vi "Search etc-hosts contents.vi"(8 "error in (no error)":errorcluster, 10 "hostname":string, 11 "/etc/hosts contents":string) -> (0 "error out":errorcluster, 3 "addresses":refnum<class "Generic Network Address.lvclass">[](array[class]))   [LabVIEW 2020, in "NI_WFCN.lvlib" / "Hostname Network Address.lvclass"]
doc: "FInd all definitions of the specified hostname in an already-read-from-disk /etc/hosts file."
uses:
  <vilib>/net/WFCN/Addressing/Hostname Network Address/Hostname Network Address.lvclass
  <vilib>/net/WFCN/Addressing/Generic Network Address/Generic Network Address.lvclass
  <vilib>/net/WFCN/Addressing/IPv4 Network Address/IPv4 Network Address.lvclass/IPv4 Network Address.ctl
  <vilib>/net/WFCN/Addressing/Generic Network Address/Generic Network Address.lvclass/Generic Network Address.ctl
  <vilib>/net/WFCN/Addressing/Hostname Network Address/Hostname Network Address.lvclass/Hostname Network Address.ctl
  <vilib>/net/WFCN/Addressing/Hostname Network Address/Create from string.vi
  <vilib>/net/WFCN/Utility/Is IPv4 address.vi
  <vilib>/net/WFCN/Addressing/IPv4 Network Address/Create from U32.vi
  <vilib>/net/WFCN/Addressing/Generic Network Address/Create for unparsable.vi
  <vilib>/net/WFCN/Utility/Is hostname mDNS.vi
  <vilib>/dlg_ctls.llb/Space Constant.vi
  <vilib>/net/WFCN/Addressing/IPv4 Network Address/IPv4 Network Address.lvclass
  e:/builds/penguin/labview/branches/2020/dev/dist/vi.lib/net/WFCN/Addressing/Generic Network Address/Generic Network Address.lvclass
  <vilib>/net/WFCN/Addressing/mDNS Hostname Network Address/mDNS Hostname Network Address.lvclass
  e:/builds/penguin/labview/branches/2020/dev/dist/vi.lib/net/WFCN/Addressing/Hostname Network Address/Hostname Network Address.lvclass
  <vilib>/Utility/error.llb/Error Cluster From Error Code.vi
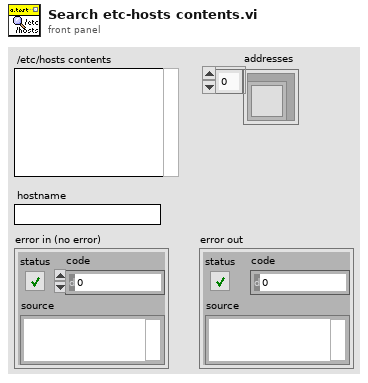
[diagram p1: front panel]
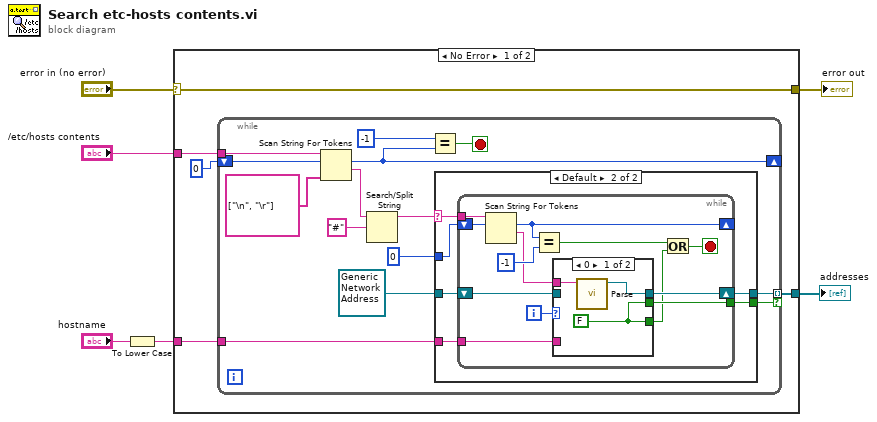
[diagram p0: block diagram]
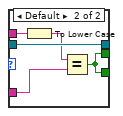
[diagram p3: hidden frame]
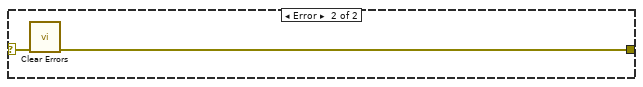
[diagram p4: hidden frame]
diagram:
  n1 = To Lower Case(string="hostname") -> (all lower case string=w1:string)
  n2 = case shown="No Error" "error in (no error)" {
    selector: "error in (no error)" -> [w9 w55]
    tunnel: [w9 w54] -> w4
    tunnel: "/etc/hosts contents" -> [w11 _]
    tunnel: w1 -> [w8 _]
    tunnel: [w7 _] -> w3
    frame No Error {
      n3 = while {
        shift-right: [w22] -> _
        shift-left: 0 ("offset past token") -> [w23]
        tunnel: w11 -> [w25]
        tunnel: w8 -> [w16]
        tunnel: [w15] -> w7 mode=indexing if=w13
        stop <- w20 stop-if-true
        n4 = Scan String For Tokens(6:string[] ["\n", "\r"], 8:w23, 9:w25) -> (1:w19:string, 2:w22:i32)  [unwired: 3 in, 2 out]
        n5 = Search/Split String(string=w19, search string/char (-)="#") -> (substring before match=w12:string)  [unwired: 1 in, 2 out]
        n6 = Equal?(x=-1 ("y"), y=w22) -> (x = y?=w20:bool)
        n7 = case shown="Default" w12 {
          selector: w12 -> [_ w27]
          tunnel: 0 ("offset past token") -> [_ w32]
          tunnel: w16 -> [_ w31]
          tunnel: [w26 w30] -> w15
          tunnel: refnum<class "Generic Network Address.lvclass"> refnum ("Network Address.lvclass") -> [w26 w29]
          tunnel: [_ w28] -> w13
          frame "" {
          }
          frame Default {
            n8 = while {
              tunnel: w27 -> [w45]
              shift-right: [w42] -> _
              shift-left: w32 -> [w44]
              tunnel: w31 -> [w38]
              shift-right: [w37] -> w30
              shift-left: w29 -> [w36]
              tunnel: [w39] -> w28
              i -> [w40]
              stop <- w33 stop-if-true
              n9 = Scan String For Tokens(8:w44, 9:w45) -> (1:w41:string, 2:w42:i32)  [unwired: 4 in, 2 out]
              n10 = Equal?(x=w42, y=-1) -> (x = y?=w35:bool)
              n11 = case shown="0" w40 {
                tunnel: w41 -> [w48 w50]
                tunnel: [w46 w52] -> w39
                tunnel: w38 -> [_ w53]
                tunnel: [w47 w51] -> w37
                tunnel: w36 -> [_ w51]
                tunnel: [w46 w52] -> w34
                frame 0 {
                  w46 = FALSE
                  n12 = call <vilib>:"Parse.vi"("address string"=w48) -> ("address"=w47:refnum<class "Generic Network Address.lvclass">)  [unwired: 10 in]
                }
                frame Default {
                  n13 = To Lower Case(string=w50) -> (all lower case string=w49:string)
                  n14 = Equal?(x=w49, y=w53) -> (x = y?=w52:bool)
                }
              }
              n15 = Or(x=w35, y=w34) -> (x .or. y?=w33:bool)
            }
          }
        }
      }
    }
    frame Error {
      n16 = call <vilib>:"Clear Errors.vi"("error in (no error)"=w55) -> ("error out"=w54:errorcluster)  [unwired: 5 in, 1 out]
    }
  }
  "error out" <- w4
  "addresses" <- w3
